vi "VL6180 Init.vi"(8 "Error In":errorcluster, 9 "I2C Slave Address (0)":u8=41 format="%x", 10 "I2C Channel":u8=1, 11 "LINX Resource":T2) -> (0 "Error Out":errorcluster, 3 "VL6180 Resource":T1 {"I2C Slave Address" format="%02x"})   [LabVIEW 2014]
uses:
  <vilib>/MakerHub/LINX/Private/Type Defs/LINX Ref.ctl
  <vilib>/MakerHub/LINX/Private/Type Defs/Platform.ctl
  <vilib>/MakerHub/LINX/Private/Type Defs/Interface.ctl
  <vilib>/MakerHub/LINX/Private/Device/Type Defs/LINX Device Config.ctl
  <vilib>/MakerHub/LINX/Private/Device/Type Defs/TCP Config.ctl
  <vilib>/MakerHub/LINX/Private/Device/Type Defs/Channels.ctl
  Type Defs/VL6180 Resource.ctl
  Type Defs/VL6180X DEFS.ctl
  <vilib>/MakerHub/LINX/LMH-LINX.lvlib
  <vilib>/MakerHub/LINX/Private/Device/Device.lvlib
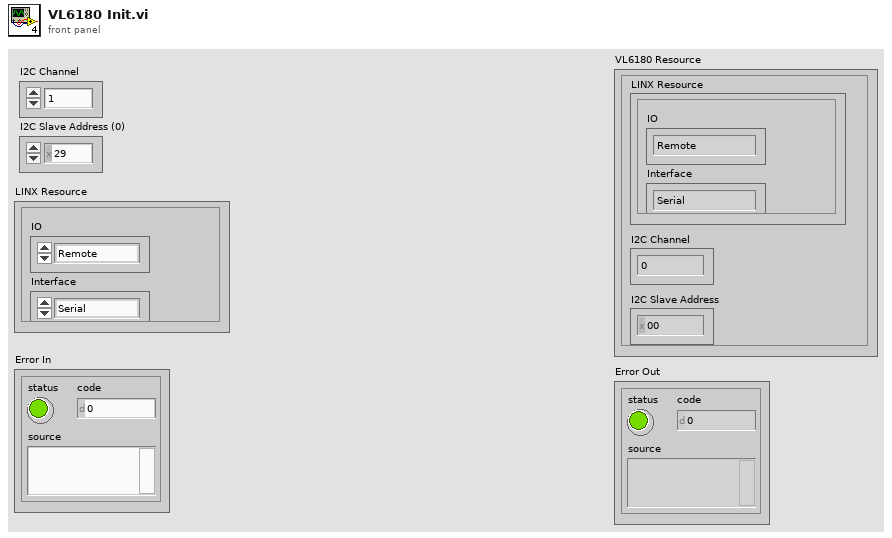
[diagram p1: front panel]
types:
  T1 = typedef "VL6180 Resource.ctl" = cluster{"LINX Resource":T2, "I2C Channel":u8, "I2C Slave Address":u8}
  T2 = typedef "LMH-LINX.lvlib/LINX Ref.ctl" = cluster{"IO":T3, "Interface":T4, "LINX Device Config":T5}
  T3 = typedef "LMH-LINX.lvlib/Platform.ctl" = enum16{"Remote", "Local"}
  T4 = typedef "LMH-LINX.lvlib/Interface.ctl" = enum16{"Serial", "TCP"}
  T5 = typedef "LMH-LINX.lvlib/Device.lvlib/LINX Device Config.ctl" = cluster{"Interface":T4, "COM Port":refnum<visa-resource-name>, "TCP Configuration":T6, "Device Family":u8, "Device ID":u8, "Device Name":string, "TCP Ref":refnum<k5>, "Channels":T7}
  T6 = typedef "LMH-LINX.lvlib/Device.lvlib/TCP Config.ctl" = cluster{"IP Address":string, "Port":u16}
  T7 = typedef "LMH-LINX.lvlib/Channels.ctl" = cluster{"DI":u8[], "DO":u8[], "AI":u8[], "AO":u8[], "PWM":u8[], "QE":u8[], "UART":u8[], "I2C 2":u8[], "SPI":u8[], "CAN":u8[], "Servo":u8[], "AI Ref (V)":dbl, "AI Resolution (Bits)":u8, "AO Ref (V)":dbl, "AO Resolution (Bits)":u8}
  T8 = typedef "VL6180X DEFS.ctl" = u16
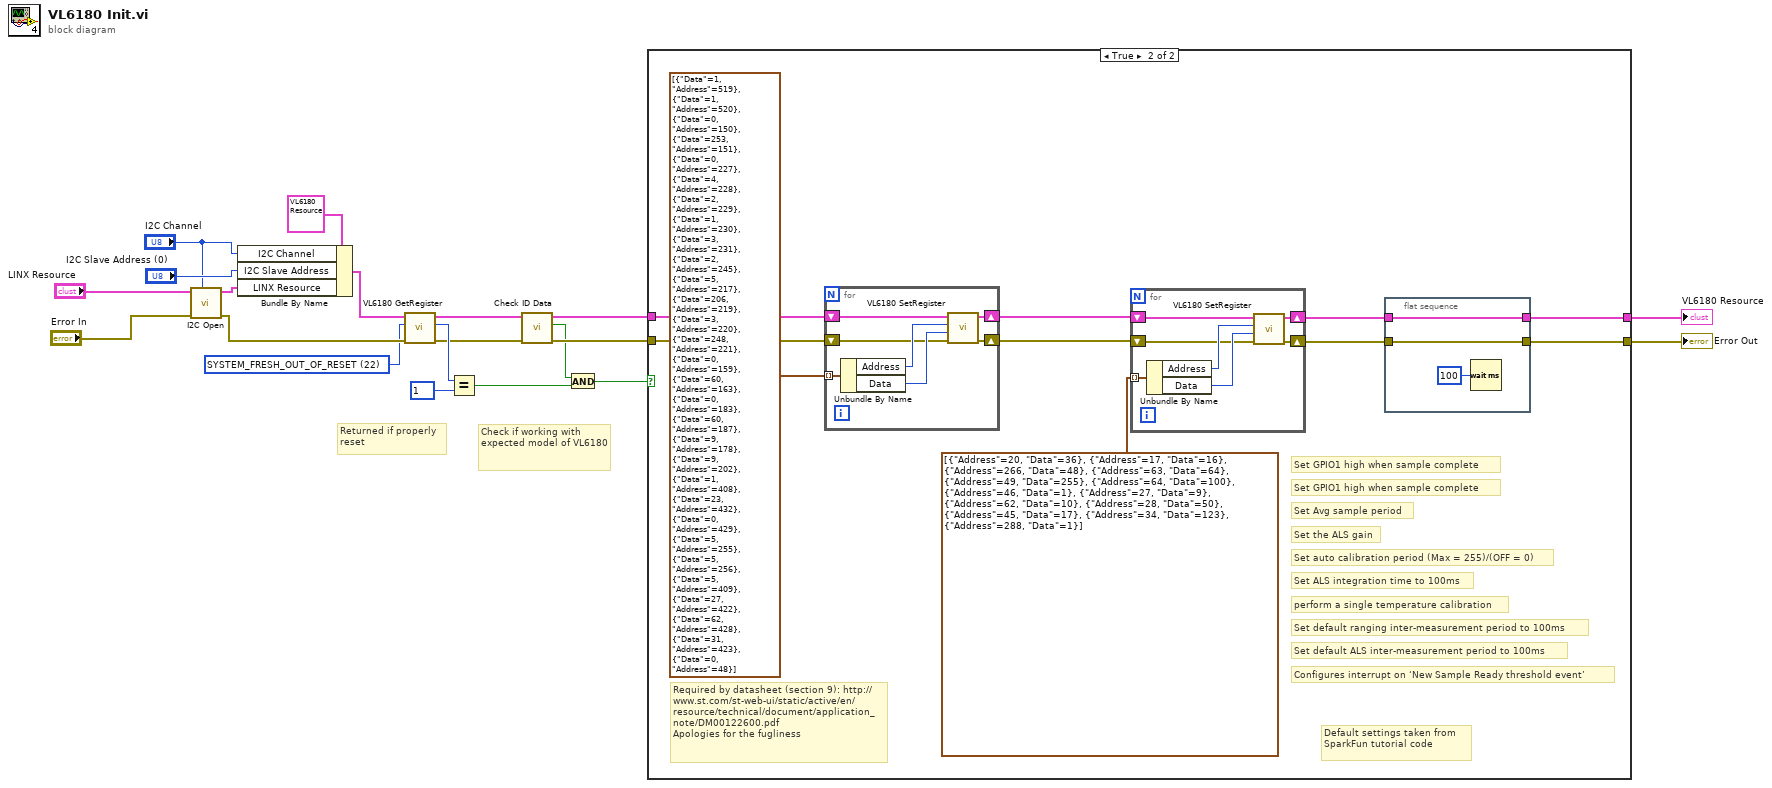
[diagram p0: block diagram]
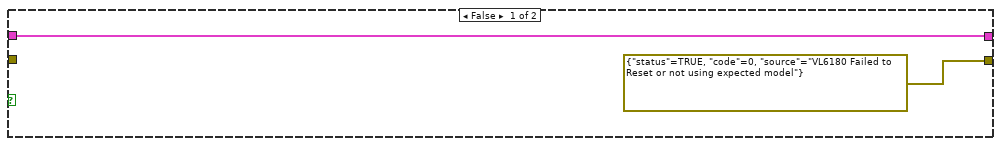
[diagram p2: hidden frame]
diagram:
  w15 = T8 22 items=["IDENTIFICATION_MODEL_ID"=0, "IDENTIFICATION_MODEL_REV_MAJOR"=1, "IDENTIFICATION_MODEL_REV_MINOR"=2, "IDENTIFICATION_MODULE_REV_MAJOR"=3, "IDENTIFICATION_MODULE_REV_MINOR"=4, "IDENTIFICATION_DATE"=6, "IDENTIFICATION_TIME"=8, "SYSTEM_MODE_GPIO0"=16, "SYSTEM_MODE_GPIO1"=17, "SYSTEM_HISTORY_CTRL"=18, "SYSTEM_INTERRUPT_CONFIG_GPIO"=20, "SYSTEM_INTERRUPT_CLEAR"=21, "SYSTEM_FRESH_OUT_OF_RESET"=22, "SYSTEM_GROUPED_PARAMETER_HOLD"=23, "SYSRANGE_START"=24, "SYSRANGE_THRESH_HIGH"=25, "SYSRANGE_THRESH_LOW"=26, "SYSRANGE_INTERMEASUREMENT_PERIOD"=27, "SYSRANGE_MAX_CONVERGENCE_TIME"=28, "SYSRANGE_CROSSTALK_COMPENSATION_RATE"=30, "SYSRANGE_CROSSTALK_VALID_HEIGHT"=33, "SYSRANGE_EARLY_CONVERGENCE_ESTIMATE"=34, "SYSRANGE_PART_TO_PART_RANGE_OFFSET"=36, "SYSRANGE_RANGE_IGNORE_VALID_HEIGHT"=37, "SYSRANGE_RANGE_IGNORE_THRESHOLD"=38, "SYSRANGE_MAX_AMBIENT_LEVEL_MULT"=44, "SYSRANGE_RANGE_CHECK_ENABLES"=45, "SYSRANGE_VHV_RECALIBRATE"=46, "SYSRANGE_VHV_REPEAT_RATE"=49, "SYSALS_START"=56, "SYSALS_THRESH_HIGH"=58, "SYSALS_THRESH_LOW"=60, "SYSALS_INTERMEASUREMENT_PERIOD"=62, "SYSALS_ANALOGUE_GAIN"=63, "SYSALS_INTEGRATION_PERIOD"=64, "RESULT_RANGE_STATUS"=77, "RESULT_ALS_STATUS"=78, "RESULT_INTERRUPT_STATUS_GPIO"=79, "RESULT_ALS_VAL"=80, "RESULT_HISTORY_BUFFER"=82, "RESULT_RANGE_VAL"=98, "RESULT_RANGE_RAW"=100, "RESULT_RANGE_RETURN_RATE"=102, "RESULT_RANGE_REFERENCE_RATE"=104, "RESULT_RANGE_RETURN_SIGNAL_COUNT"=108, "RESULT_RANGE_REFERENCE_SIGNAL_COUNT"=112, "RESULT_RANGE_RETURN_AMB_COUNT"=116, "RESULT_RANGE_REFERENCE_AMB_COUNT"=120, "RESULT_RANGE_RETURN_CONV_TIME"=124, "RESULT_RANGE_REFERENCE_CONV_TIME"=128, "READOUT_AVERAGING_SAMPLE_PERIOD"=266, "FIRMWARE_BOOTUP"=281, "FIRMWARE_RESULT_SCALER"=288, "I2C_SLAVE_DEVICE_ADDRESS"=530, "INTERLEAVED_MODE_ENABLE"=675] ("VL6180X Constants")
  # "Check if working with expected model of VL6180"
  # "Returned if properly\nreset"
  n1 = call <vilib>:"I2C Open.vi"("I2C Channel (0)"="I2C Channel", "Error In"="Error In", "LINX Resource"="LINX Resource") -> ("Error Out"=w20:errorcluster, "LINX Resource"=w12:T2)  [unwired: 7 in]
  n2 = Bundle By Name(cluster=T1 {"LINX Resource"={"IO"=enum."Remote", "Interface"=enum."Serial", "LINX Device Config"={"Interface"=enum."Serial", "COM Port"="", "TCP Configuration"={"IP Address"="", "Port"=0}, "Device Family"=0, "Device ID"=0, "Device Name"="", "TCP Ref"=refnum, "Channels"={"DI"=[], "DO"=[], "AI"=[], "AO"=[], "PWM"=[], "QE"=[], "UART"=[], "I2C 2"=[], "SPI"=[], "CAN"=[], "Servo"=[], "AI Ref (V)"=0.0, "AI Resolution (Bits)"=0, "AO Ref (V)"=0.0, "AO Resolution (Bits)"=0}}}, "I2C Channel"=0, "I2C Slave Address"=0} ("VL6180 Resource"), "I2C Channel"="I2C Channel", "I2C Slave Address"="I2C Slave Address (0)", "LINX Resource"=w12) -> (w11:T1)
  n3 = call "VL6180 GetRegister.vi"("error in"=w20, "VL6180X Constants"=w15, "VL6180 Resource"=w11) -> ("error out"=w6:errorcluster, "Data out"=w14:u8, "VL6180 Resource"=w7:T1)  [unwired: 6 in]
  n4 = Equal?(x=w14, y=u8 1 ("Data 2")) -> (x = y?=w4:bool)
  n5 = call "Check ID Data.vi"("Error In"=w6, "VL6180 Resource"=w7) -> ("Error Out"=w8:errorcluster, "Same Model?"=w5:bool, "VL6180 Resource"=w9:T1)  [unwired: 7 in]
  n6 = And(x=w5, y=w4) -> (x .and. y?=w2:bool)
  n7 = case shown="True" w2 {
    tunnel: w8 -> [_ w30]
    tunnel: [errorcluster {"status"=TRUE, "code"=0, "source"="VL6180 Failed to Reset or not using expected model"} ("Error Out") w23] -> w16
    tunnel: w9 -> [w21 w32]
    tunnel: [w21 w24] -> w3
    frame False {
    }
    frame True {
      # "Default settings taken from SparkFun tutorial code"
      # "Configures interrupt on ‘New Sample Ready threshold event’"
      # "Set default ALS inter-measurement period to 100ms"
      # "Set default ranging inter-measurement period to 100ms"
      # "perform a single temperature calibration"
      # "Set ALS integration time to 100ms"
      # "Set auto calibration period (Max = 255)/(OFF = 0)"
      # "Set the ALS gain"
      # "Set Avg sample period"
      # "Set GPIO1 high when sample complete"
      # "Set GPIO1 high when sample complete"
      # "Required by datasheet (section 9): http://www.st.com/st-web-ui/static/active/en/resource/technical/document/application_note/DM00122600.pdf\nApologies for the fugliness"
      n8 = for {
        tunnel: cluster{"Data":u8, "Address":u16}[] [{"Data"=1, "Address"=519}, {"Data"=1, "Address"=520}, {"Data"=0, "Address"=150}, {"Data"=253, "Address"=151}, {"Data"=0, "Address"=227}, {"Data"=4, "Address"=228}, {"Data"=2, "Address"=229}, {"Data"=1, "Address"=230}, {"Data"=3, "Address"=231}, {"Data"=2, "Address"=245}, {"Data"=5, "Address"=217}, {"Data"=206, "Address"=219}, {"Data"=3, "Address"=220}, {"Data"=248, "Address"=221}, {"Data"=0, "Address"=159}, {"Data"=60, "Address"=163}, {"Data"=0, "Address"=183}, {"Data"=60, "Address"=187}, {"Data"=9, "Address"=178}, {"Data"=9, "Address"=202}, {"Data"=1, "Address"=408}, {"Data"=23, "Address"=432}, {"Data"=0, "Address"=429}, {"Data"=5, "Address"=255}, {"Data"=5, "Address"=256}, {"Data"=5, "Address"=409}, {"Data"=27, "Address"=422}, {"Data"=62, "Address"=428}, {"Data"=31, "Address"=423}, {"Data"=0, "Address"=48}] -> [w48] mode=indexing
        shift-right: [w43] -> w27
        shift-left: w30 -> [w45]
        shift-right: [w44] -> w28
        shift-left: w32 -> [w49]
        n9 = Unbundle By Name(w48) -> ("Address"=w47:u16, "Data"=w46:u8)
        n10 = call "VL6180 SetRegister.vi"("error in (no error)"=w45, "Data in"=w46, "Address"=w47, "VL6180 Resource"=w49) -> ("error out"=w43:errorcluster, "VL6180 Resource"=w44:T1)  [unwired: 6 in]
      }
      n11 = for {
        tunnel: cluster{"Address":T8, "Data":u8}[] [{"Address"=20, "Data"=36}, {"Address"=17, "Data"=16}, {"Address"=266, "Data"=48}, {"Address"=63, "Data"=64}, {"Address"=49, "Data"=255}, {"Address"=64, "Data"=100}, {"Address"=46, "Data"=1}, {"Address"=27, "Data"=9}, {"Address"=62, "Data"=10}, {"Address"=28, "Data"=50}, {"Address"=45, "Data"=17}, {"Address"=34, "Data"=123}, {"Address"=288, "Data"=1}] -> [w41] mode=indexing
        shift-right: [w36] -> w25
        shift-left: w27 -> [w38]
        shift-right: [w37] -> w26
        shift-left: w28 -> [w42]
        n12 = Unbundle By Name(w41) -> ("Address"=w40:T8, "Data"=w39:u8)
        n13 = call "VL6180 SetRegister.vi"("error in (no error)"=w38, "Data in"=w39, "Address"=w40, "VL6180 Resource"=w42) -> ("error out"=w36:errorcluster, "VL6180 Resource"=w37:T1)  [unwired: 6 in]
      }
      n14 = flat-sequence {
        tunnel: w26 -> [w35]
        tunnel: w25 -> [w34]
        tunnel: [w35] -> w24
        tunnel: [w34] -> w23
        frame #0 {
          n15 = Wait (ms)(milliseconds to wait=u32 100) -> ()  [unwired: 1 out]
        }
      }
    }
  }
  "Error Out" <- w16
  "VL6180 Resource" <- w3
